vi "Read Tobj.vi"(8 "error in (no error)":errorcluster, 11 "humData in":refnum<class "humData.lvclass">) -> (0 "error out":errorcluster, 2 "Tobj":dbl, 3 "humData out":refnum<class "humData.lvclass">)   [LabVIEW 2014, in "humData.lvclass"]
uses:
  humData.lvclass
  humData.lvclass/humData.ctl
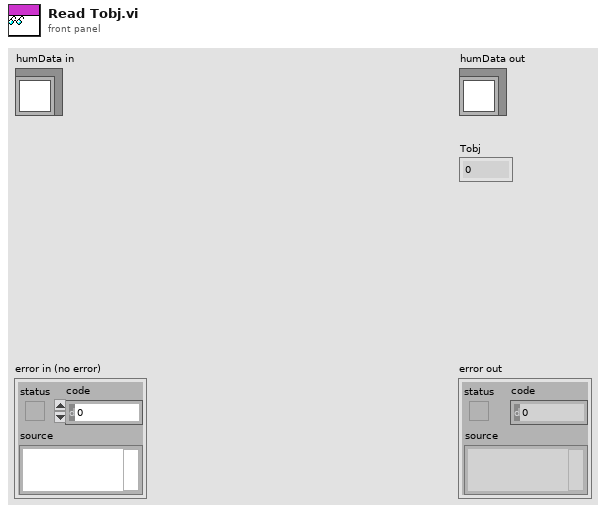
[diagram p1: front panel]
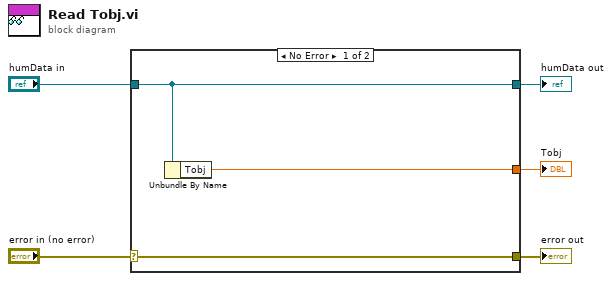
[diagram p0: block diagram]
diagram:
  n1 = case shown="No Error" "error in (no error)" {
    selector: "error in (no error)" -> [w8 w9]
    tunnel: [w8 w9] -> w4
    tunnel: [w7 w10] -> w2
    tunnel: "humData in" -> [w7 w10]
    tunnel: [w6 _] -> w1
    frame No Error {
      n2 = Unbundle By Name(w7) -> ("Tobj"=w6:dbl)
    }
    frame Error {
    }
  }
  "error out" <- w4
  "humData out" <- w2
  "Tobj" <- w1
